vi "Вывод температуры.vi"() -> ()   [LabVIEW 2017]
doc: "This VI is used as a subVI in the Temperature System exercise in the LabVIEW Basics I course."
panel:
  in  "Return":bool
  out "Температура":dbl(graph)
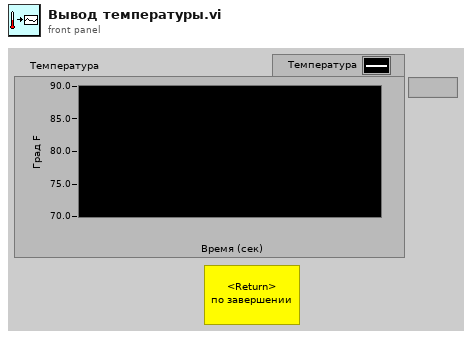
[diagram p1: front panel]
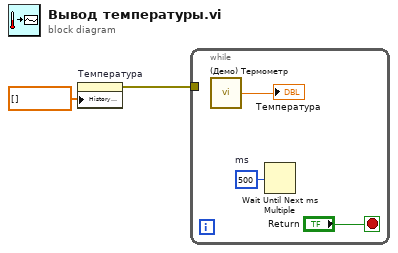
[diagram p0: block diagram]
diagram:
  n1 = property on="Температура" class="WFChart (strict)"("History Data"=dbl[] []) -> (error out=w1:errorcluster)  [unwired: 2 in, 1 out]
  n2 = while {
    tunnel: w1 -> [_]
    stop <- "Return" stop-if-true
    w4 = u32 500  # ms
    n3 = call "(Демо) Термометр.vi"() -> ("Температура"=→"Температура":dbl)  [unwired: 1 in]
    n4 = Wait Until Next ms Multiple(millisecond multiple=w4) -> ()  [unwired: 1 out]
  }
